vi "Producer Consumer Data.vi"() -> ()   [LabVIEW 2012]
doc: "该模板用于创建生产者／消费者模式的应用程序。该模板可用于执行诸如数据分析的数据处理，或者在以不均匀速率产生数据的数据源中（如触发采集），当数据可用时对数据进行分析。"
panel:
  out "队列积压空间":i32(slide) scale=0.0..100.0
  in  "消费者循环中的“等待（毫秒）”":u32(slide) scale=0.0..10000.0
  out "出队数据":string="元素"
  in  "待入队数据":string="元素"
  in  "入队数据":bool
  in  "停止":bool
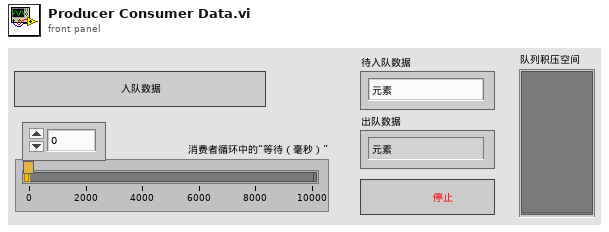
[diagram p1: front panel]
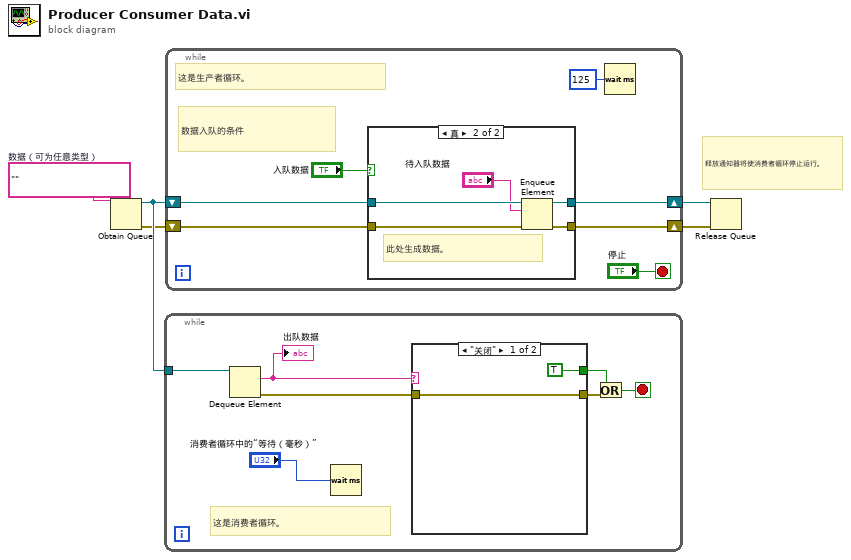
[diagram p0: block diagram]
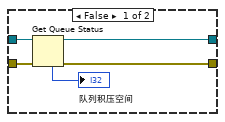
[diagram p3: hidden frame]
diagram:
  w1 = ""  # 数据（可为任意类型）
  # "释放通知器将使消费者循环停止运行。"
  n1 = Obtain Queue ("获取队列引用")(element data type=w1) -> (queue out=w5:refnum<queue>, error out=w4:errorcluster)  [unwired: 4 in, 1 out]
  n2 = while {
    tunnel: w5 -> [w12]
    stop <- w9 stop-if-true
    # "这是消费者循环。"
    n3 = Dequeue Element ("元素出队列")(queue=w12) -> (element=w6:string, error out=w11:errorcluster)  [unwired: 2 in, 2 out]
    "出队数据" <- w6
    n4 = Wait (ms) ("等待(ms)")(milliseconds to wait="消费者循环中的“等待（毫秒）”") -> ()  [unwired: 1 out]
    n5 = case shown="\"关闭\"" w6 {
      tunnel: [TRUE _] -> w8
      tunnel: [w13 w15] -> w10
      tunnel: w11 -> [w13 w15]
      frame "关闭" {
      }
      frame Default {
      }
    }
    n6 = Or ("或")(x=w8, y=w10) -> (x .or. y?=w9:bool)
  }
  n7 = while {
    shift-right: [w18] -> w2
    shift-left: w4 -> [w19]
    shift-right: [w20] -> w3
    shift-left: w5 -> [w21]
    stop <- "停止" stop-if-true
    # "数据入队的条件"
    # "这是生产者循环。"
    n8 = case shown="真" "入队数据" {
      tunnel: w21 -> [w25 w32]
      tunnel: [w24 w31] -> w20
      tunnel: w19 -> [w27 w30]
      tunnel: [w26 w29] -> w18
      frame False {
        n9 = Get Queue Status ("获取队列状态")(queue=w25, error in (no error)=w27) -> (queue out=w24:refnum<queue>, error out=w26:errorcluster, # elements in queue=→"队列积压空间":i32)  [unwired: 1 in, 5 out]
      }
      frame True {
        # "此处生成数据。"
        n10 = Enqueue Element ("元素入队列")(queue=w32, element="待入队数据", error in (no error)=w30) -> (queue out=w31:refnum<queue>, error out=w29:errorcluster)  [unwired: 1 in, 1 out]
      }
    }
    n11 = Wait (ms) ("等待(ms)")(milliseconds to wait=u32 125 ("等待时间（毫秒）")) -> ()  [unwired: 1 out]
  }
  n12 = Release Queue ("释放队列引用")(queue=w3, error in (no error)=w2) -> ()  [unwired: 1 in, 3 out]
